vi "G4BaseTemplate_Singleton_6x8x6_GetInstance.vi"(0 "reference in":refnum<class "G4BaseTemplate_Singleton_6x8x6.lvclass"> caption="This control should only be used when\na sub class is inheriting this class", 5 "Error In":errorcluster) -> (12 "ObjectQueueName":string caption="This queue name could be used to destroy\nthe named queue that is used to hold the\nreference in the clean up.", 14 "reference out":refnum<class "G4BaseTemplate_Singleton_6x8x6.lvclass">, 15 "NewObjectCreated":bool, 16 "DVRRefOut":refnum<data-value>, 19 "Error Out":errorcluster)   [LabVIEW 2020, in "G4BaseTemplate_Singleton_6x8x6.lvclass"]
uses:
  G4BaseTemplate_Singleton_6x8x6.lvclass
  ObjectAttributes.ctl
  G4BaseTemplate_Singleton_6x8x6.lvclass/G4BaseTemplate_Singleton_6x8x6.ctl
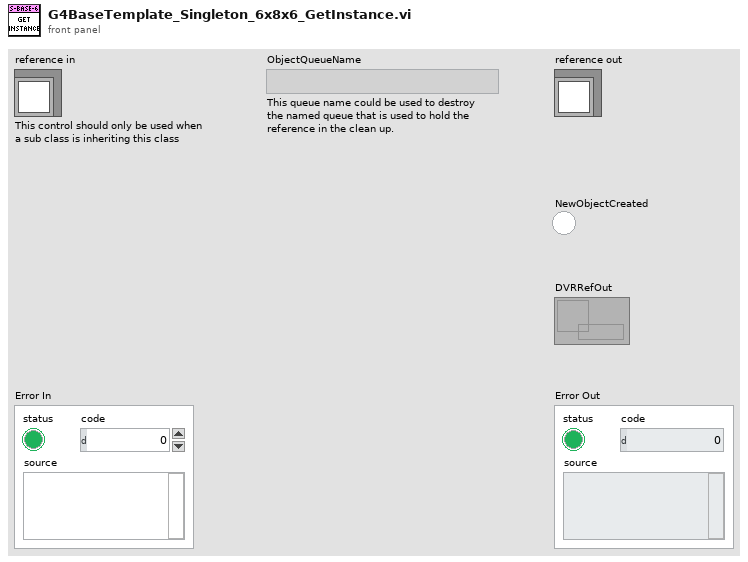
[diagram p1: front panel]
types:
  T1 = enum16{"Create or look up existing", "Look up existing"}
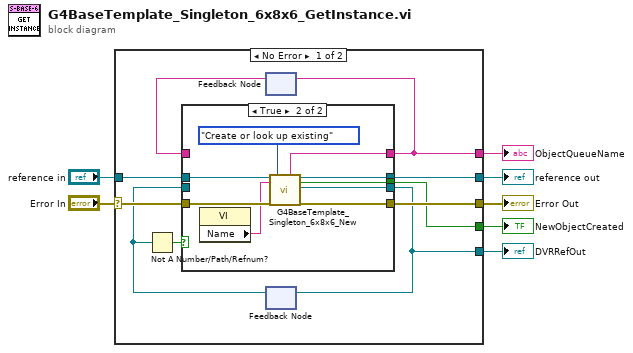
[diagram p0: block diagram]
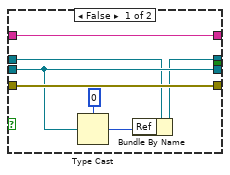
[diagram p2: hidden frame]
diagram:
  n1 = case shown="No Error" "Error In" {
    selector: "Error In" -> [w16 w35]
    tunnel: [w17 w34] -> w7
    tunnel: [w15 w35] -> w5
    tunnel: "reference in" -> [w14 w34]
    tunnel: [w13 _] -> w3
    tunnel: [w12 _] -> w2
    tunnel: [w9 _] -> w1
    frame No Error {
      n2 = feedback #1() -> (w8:string)  [unwired: 1 in]
      n3 = feedback #2() -> (w10:refnum<data-value>)  [unwired: 1 in]
      n4 = Not A Number/Path/Refnum?(number/path/refnum=w10) -> (NaN/Path/Refnum?=w11:bool)
      n5 = case shown="True" w11 {
        tunnel: [w19 w33] -> w17
        tunnel: w16 -> [w24 w32]
        tunnel: [w24 w31] -> w15
        tunnel: w14 -> [w18 w29]
        tunnel: [_ w28] -> w13
        tunnel: [w23 w26] -> w9
        tunnel: [w20 w25] -> w12
        tunnel: w10 -> [w20 _]
        tunnel: w8 -> [w23 _]
        frame False {
          n6 = Type Cast(type=u32 0, x=w20) -> (*(type *) &x=w21:u32)
          n7 = Bundle By Name(cluster=w18, "Ref"=w21) -> (w19:refnum<class "G4BaseTemplate_Singleton_6x8x6.lvclass">)
        }
        frame True {
          n8 = property class="VI"() -> ("Name"=w30:string)  [unwired: 2 in, 2 out]
          n9 = call "G4BaseTemplate_Singleton_6x8x6_New.vi"("reference in"=w29, "Object name"=w30, "Error In"=w32, "CreateMethod(Create or look up existing)"=T1."Create or look up existing") -> ("ObjectQueueName"=w26:string, "reference out"=w33:refnum<class "G4BaseTemplate_Singleton_6x8x6.lvclass">, "NewObjectCreated"=w28:bool, "DVRRefOut"=w25:refnum<data-value>, "Error Out"=w31:errorcluster)  [unwired: 11 in]
        }
      }
      n10 = feedback-in #1(w9) -> ()
      n11 = feedback-in #2(w12) -> ()
    }
    frame Error {
    }
  }
  "reference out" <- w7
  "Error Out" <- w5
  "NewObjectCreated" <- w3
  "DVRRefOut" <- w2
  "ObjectQueueName" <- w1
